vi "Get port Status.vi"(8 "error in (no error)":errorcluster, 10 "Puerto":dbl, 11 "Simulado in":refnum<class "Simulado.lvclass">) -> (0 "error out":errorcluster, 3 "Simulado out":refnum<class "Simulado.lvclass">)   [LabVIEW 2020, in "Simulado.lvclass"]
uses:
  Simulado.lvclass
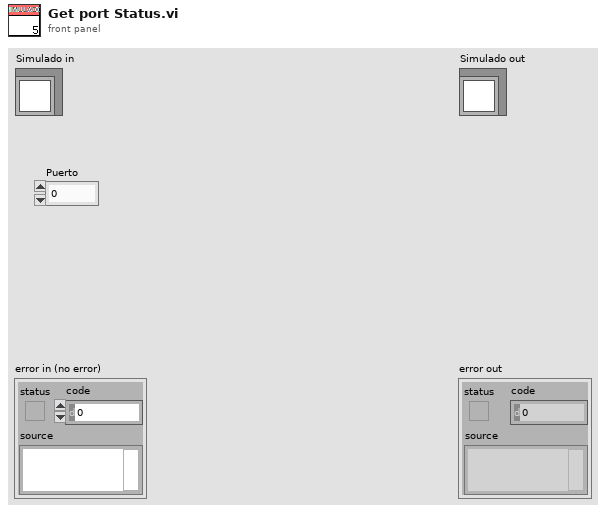
[diagram p1: front panel]
types:
  T1 = typedef "Serial Device.lvclass/serial device brand.ctl" = string
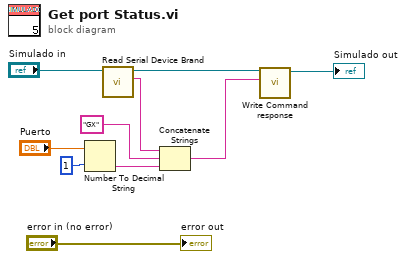
[diagram p0: block diagram]
diagram:
  n1 = Number To Decimal String(number="Puerto", width (-)=i16 1) -> (decimal integer string=w4:string)
  n2 = call-dynamic "Read Serial Device Brand.vi"("Serial Device in"="Simulado in") -> ("Serial Device Brand"=w5:T1, "Serial Device out"=w9:refnum<class "Simulado.lvclass">)  [unwired: 8 in, 1 out]
  n3 = Concatenate Strings(w5, "GX" ("string"), w4) -> (w2:string)
  n4 = call-dynamic "Write Command response.vi"("Command response"=w2, "Simulado in"=w9) -> ("Simulado out"=→"Simulado out":refnum<class "Simulado.lvclass">)  [unwired: 8 in, 1 out]
  "error out" <- "error in (no error)"
